vi "Create Parameter For Each Word.vi"(8 "error in":errorcluster, 11 "number of words":u16) -> (0 "error out":errorcluster, 3 "parameters":T2(array[cluster]))   [LabVIEW 2020, in "AIM MIL-STD 1553 Shared.lvlib"]
uses:
  Parameter Definition.ctl
  AIM MIL-STD 1553 Shared.lvlib
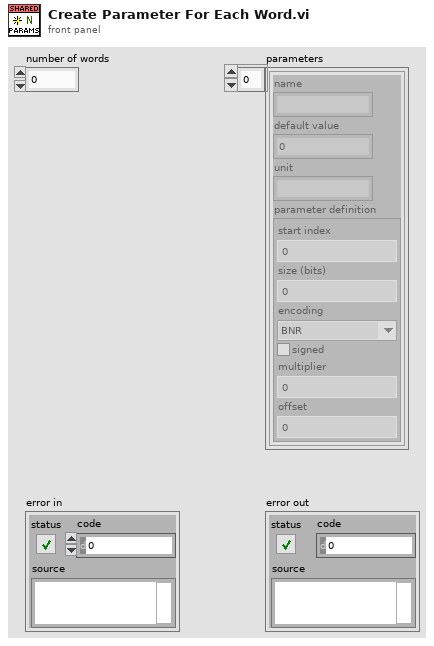
[diagram p1: front panel]
types:
  T1 = typedef "AIM MIL-STD 1553 Shared.lvlib/Parameter Definition.ctl" = cluster{"start index":i32, "size (bits)":i32, "encoding":enum16{"BNR", "BCD", "Discrete"}, "signed":bool, "multiplier":dbl, "offset":dbl}
  T2 = cluster{"name":string, "default value":dbl, "unit":string, "parameter definition":T1}[]
  T3 = cluster{"name":string, "default value":dbl, "unit":string, "parameter definition":T1}
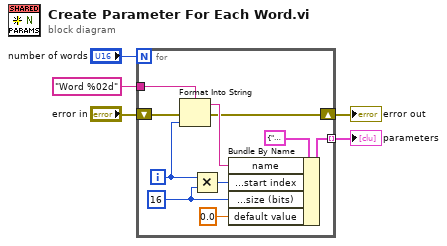
[diagram p0: block diagram]
diagram:
  n1 = for {
    N: "number of words" -> [_]
    tunnel: [w8] -> w3 mode=indexing
    shift-right: [w9] -> w5
    shift-left: "error in" -> [w10]
    tunnel: "Word %02d" ("format string") -> [w7]
    i -> [w13]
    w12 = 16 ("y")
    n2 = Format Into String(format string=w7, error in=w10, w13) -> (resulting string=w15:string, error out=w9:errorcluster)  [unwired: 1 in]
    n3 = Multiply(x=w13, y=w12) -> (x*y=w14:i32)
    n4 = Bundle By Name(cluster=T3 {"name"="", "default value"=1.0, "unit"="", "parameter definition"={"start index"=0, "size (bits)"=16, "encoding"=enum."BNR", "signed"=FALSE, "multiplier"=1.0, "offset"=0.0}} ("definition with default value"), "name"=w15, "parameter definition.start index"=w14, "parameter definition.size (bits)"=w12, "default value"=0.0) -> (w8:T3)
  }
  "error out" <- w5
  "parameters" <- w3
